vi "test Broadcast Function Code Typedef.vi"(11 "Test Case In":refnum<class "Function Code Typedef Test.lvclass">) -> (0 "error out":errorcluster, 3 "Test Case Out":refnum<class "Function Code Typedef Test.lvclass">)   [LabVIEW 2020, in "Function Code Typedef Test.lvclass"]
uses:
  Function Code Typedef Test.lvclass
  Function Code Typedef Test.lvclass/Function Code Typedef Test.ctl
  C:/Program Files/National Instruments/LabVIEW 2026/vi.lib/Astemes/LUnit/Test Case.lvclass
  C:/Program Files/National Instruments/LabVIEW 2026/vi.lib/Astemes/LUnit/LUnit Runnable.lvclass
  D:/git/CANopen-LabVIEW/Tests/Function Code Typedef Test/Function Code Typedef Test.lvclass
  4993e8ee-a06a-463a-9684-69129f64d5ce.vi
  CANopen/Broadcast Function Code.ctl
panel:
  out "x = y?":bool
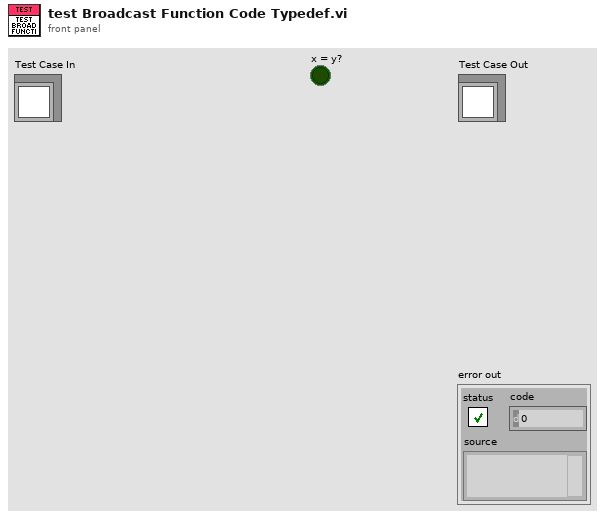
[diagram p1: front panel]
types:
  T1 = typedef "CANopen.lvlib/CANopen.lvclass/Broadcast Function Code.ctl" = map{string, i32}
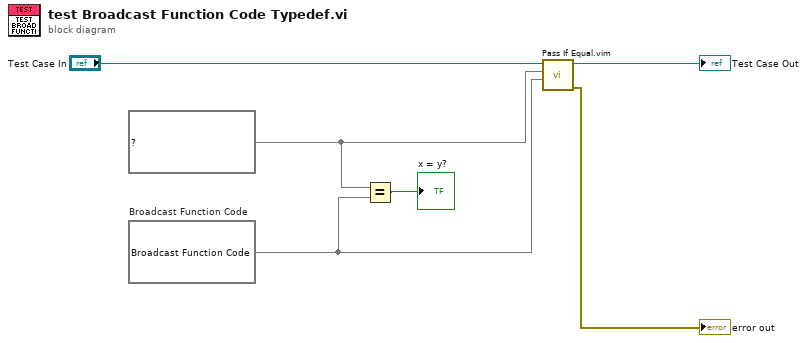
[diagram p0: block diagram]
diagram:
  w3 = map{string, i32} {"NMT"=0, "SYNC"=1, "TIME"=2} ("Function Code")
  w2 = T1 {"NMT"=0, "SYNC"=1, "TIME"=2}  # Broadcast Function Code
  n1 = Equal?(x=w3, y=w2) -> (x = y?=→"x = y?":bool)
  n2 = call "Pass If Equal.vim"("Actual"=w2, "Expected"=w3, "LUnit Test Case In"="Test Case In") -> ("error out"=→"error out":errorcluster, "LUnit Test Case Out"=→"Test Case Out":refnum<class "Function Code Typedef Test.lvclass">)  [unwired: 7 in]
